vi "WPI_UtilitiesGetCommandParams.vi"(8 "error in":errorcluster, 11 "VI in":refnum<vi>) -> (2 "Array":string[](array[string]), 3 "VI out":refnum<vi>)   [LabVIEW 2019]
uses:
  <vilib>/Utility/Data Type/NI_Data Type.lvlib
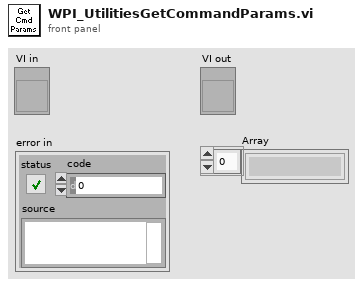
[diagram p1: front panel]
types:
  T1 = typedef "NI_Data Type.lvlib/Data Type.ctl" = enum8{"Invalid Type", "Void", "I8", "I16", "I32", "I64", "U8", "U16", "U32", "U64", "Single Float", "Double Float", "Extended Float", "Single Complex", "Double Complex", "Extended Complex", "Enum U8", "Enum U16", "Enum U32", "Enum U64", "Single Float With Unit", "Double Float With Unit", "Extended Float With Unit", "Single Complex with Unit", "Double Complex with Unit", "Extended Complex with Unit", "Boolean", "String", "Path", "Picture", "Tag", "Array", "Cluster", "Variant", "LV Variant", "Waveform", "Timestamp", "Digital Waveform", "Digital Data", "ExpressData", "Refnum", "External Data", "VI", "Poly VI", "LabVIEW Class Instance", "Fixed Point", "Set Collection", "Map Collection"}
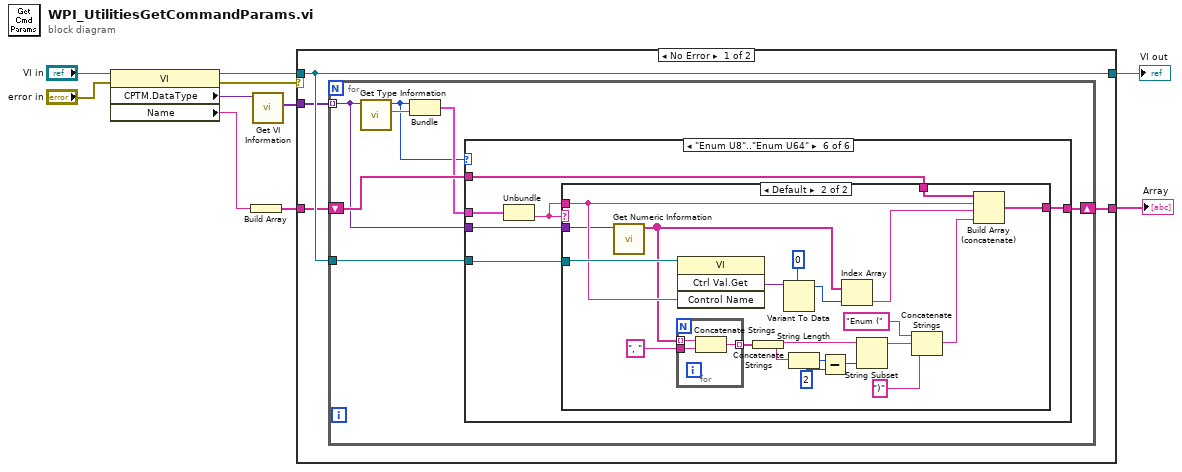
[diagram p0: block diagram]
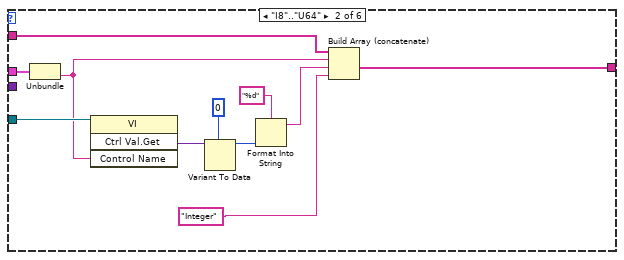
[diagram p3: hidden frame]
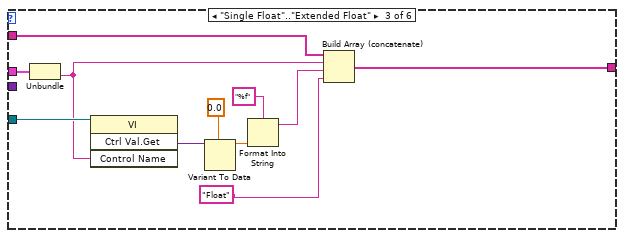
[diagram p4: hidden frame]
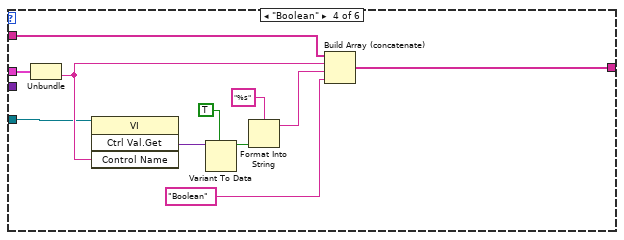
[diagram p5: hidden frame]
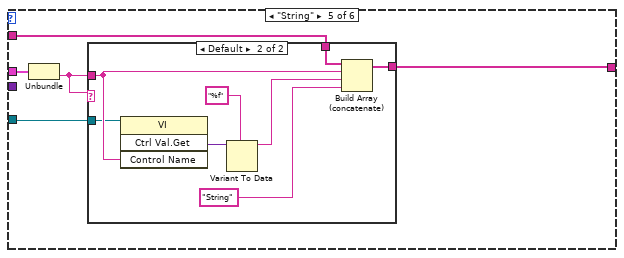
[diagram p6: hidden frame]
diagram:
  n1 = property class="VI"(reference="VI in", error in="error in") -> (reference out=w6:refnum<vi>, error out=w8:errorcluster, "CPTM.DataType"=w2:variant, "Name"=w3:string)
  n2 = Build Array(w3) -> (w4:string[])
  n3 = call <vilib>:"Get VI Information.vi"("variant"=w2) -> ("VI terminal types"=w1:variant[])  [unwired: 7 in, 3 out]
  n4 = case shown="No Error" w8 {
    tunnel: [w14 w100] -> w10
    tunnel: w6 -> [w14 w100]
    tunnel: [w13 _] -> w9
    tunnel: w4 -> [w12 _]
    tunnel: w1 -> [w11 _]
    frame No Error {
      n5 = for {
        tunnel: w14 -> [w21]
        shift-right: [w20] -> w13
        shift-left: w12 -> [w19]
        tunnel: w11 -> [w15] mode=indexing
        n6 = call <vilib>:"Get Type Information.vi"("variant"=w15) -> ("name"=w18:string, "type"=w16:T1)  [unwired: 6 in, 3 out]
        n7 = Bundle("type"=w16, "name"=w18) -> (w17:cluster{"type":T1, "name":string})  [unwired: 1 in]
        n8 = case shown="\"Enum U8\"..\"Enum U64\"" w16 {
          tunnel: w17 -> [_ w32 w43 w49 w60 w75]
          tunnel: w21 -> [_ w33 w44 w50 w59 w74]
          tunnel: [w22 w23 w34 w45 w57 w72] -> w20
          tunnel: w19 -> [w22 w24 w35 w46 w58 w73]
          tunnel: w15 -> [_ _ _ _ _ w70]
          frame "Invalid Type", Default {
          }
          frame "I8".."U64" {
            n9 = Unbundle(w32) -> ("name"=w28:string)  [unwired: 1 out]
            n10 = invoke class="VI" method="Ctrl Val.Get"(reference=w33, "Control Name"=w28) -> ("Get Control Value Variant"=w26:variant)  [unwired: 2 in, 3 out]
            n11 = Variant To Data(type=i64 0, Variant=w26) -> (data=w29:i64)  [unwired: 1 in, 1 out]
            n12 = Format Into String(format string="%d", w29) -> (resulting string=w27:string)  [unwired: 2 in, 1 out]
            n13 = Build Array (concatenate)(w24, w28, w27, "Integer" ("format string")) -> (w23:string[])
          }
          frame "Single Float".."Extended Float" {
            n14 = Unbundle(w43) -> ("name"=w39:string)  [unwired: 1 out]
            n15 = invoke class="VI" method="Ctrl Val.Get"(reference=w44, "Control Name"=w39) -> ("Get Control Value Variant"=w38:variant)  [unwired: 2 in, 3 out]
            n16 = Variant To Data(type=0.0, Variant=w38) -> (data=w40:dbl)  [unwired: 1 in, 1 out]
            n17 = Format Into String(format string="%f", w40) -> (resulting string=w37:string)  [unwired: 2 in, 1 out]
            n18 = Build Array (concatenate)(w35, w39, w37, "Float" ("format string")) -> (w34:string[])
          }
          frame "Boolean" {
            n19 = Unbundle(w49) -> ("name"=w53:string)  [unwired: 1 out]
            n20 = invoke class="VI" method="Ctrl Val.Get"(reference=w50, "Control Name"=w53) -> ("Get Control Value Variant"=w52:variant)  [unwired: 2 in, 3 out]
            n21 = Variant To Data(type=TRUE, Variant=w52) -> (data=w54:bool)  [unwired: 1 in, 1 out]
            n22 = Format Into String(format string="%s", w54) -> (resulting string=w51:string)  [unwired: 2 in, 1 out]
            n23 = Build Array (concatenate)(w46, w53, w51, "Boolean" ("format string")) -> (w45:string[])
          }
          frame "String" {
            n24 = Unbundle(w60) -> ("name"=w56:string)  [unwired: 1 out]
            n25 = case shown="Default" w56 {
              tunnel: w56 -> [_ w69]
              tunnel: w59 -> [_ w67]
              tunnel: w58 -> [w61 w63]
              tunnel: [w61 w62] -> w57
              frame "Description" {
              }
              frame Default {
                n26 = invoke class="VI" method="Ctrl Val.Get"(reference=w67, "Control Name"=w69) -> ("Get Control Value Variant"=w68:variant)  [unwired: 2 in, 3 out]
                n27 = Variant To Data(type="%f" ("format string"), Variant=w68) -> (data=w64:string)  [unwired: 1 in, 1 out]
                n28 = Build Array (concatenate)(w63, w69, w64, "String" ("format string")) -> (w62:string[])
              }
            }
          }
          frame "Enum U8".."Enum U64" {
            n29 = Unbundle(w75) -> ("name"=w71:string)  [unwired: 1 out]
            n30 = case shown="Default" w71 {
              tunnel: w71 -> [_ w81]
              tunnel: w74 -> [_ w82]
              tunnel: w73 -> [w76 w79]
              tunnel: [w76 w80] -> w72
              tunnel: w70 -> [_ w78]
              frame "Synchronization" {
              }
              frame Default {
                n31 = call <vilib>:"Get Numeric Information.vi"("variant"=w78) -> ("enum names"=w77:string[])  [unwired: 7 in, 3 out]
                n32 = for {
                  tunnel: w77 -> [w99] mode=indexing
                  tunnel: [w98] -> w84 mode=indexing
                  tunnel: ", " ("format string") -> [w97]
                  n33 = Concatenate Strings(w99, w97) -> (w98:string)
                }
                n34 = invoke class="VI" method="Ctrl Val.Get"(reference=w82, "Control Name"=w81) -> ("Get Control Value Variant"=w96:variant)  [unwired: 2 in, 3 out]
                n35 = Concatenate Strings(w84) -> (w83:string)
                n36 = Variant To Data(type=u32 0, Variant=w96) -> (data=w94:u32)  [unwired: 1 in, 1 out]
                n37 = String Length(string=w83) -> (length=w86:i32)
                n38 = Subtract(x=w86, y=u32 2) -> (x-y=w87:u32)
                n39 = Index Array(array=w77, index=w94) -> (element=w93:string)
                n40 = String Subset(string=w83, length (rest)=w87) -> (substring=w89:string)  [unwired: 1 in]
                n41 = Concatenate Strings("Enum (" ("format string"), w89, ")" ("format string")) -> (w90:string)
                n42 = Build Array (concatenate)(w79, w81, w93, w90) -> (w80:string[])
              }
            }
          }
        }
      }
    }
    frame Error {
    }
  }
  "VI out" <- w10
  "Array" <- w9
